vi "select io channels.vi"(8 "error in":errorcluster, 9 "API Loaded":string, 10 "not supported channels":refnum<class "TBM channel.lvclass">[](array[class]), 11 "io channels":refnum<class "TBM channel.lvclass">[](array[class])) -> (0 "error out":errorcluster, 3 "selected channels":refnum<class "TBM channel.lvclass">[](array[class]))   [LabVIEW 2015, in "io editor node.lvclass"]
uses:
  io editor node.lvclass
  <vilib>/NI/Tag Bus Module Framework/channel/TBM channel.lvclass
  table line.ctl
  table reference.ctl
panel:
  in  "Tab Control":enum32{"Static Configuration"}(tab)
  in  "cancel":bool
  in  "select channels":bool
  in  "channel":i32[](listbox)
  out "API Loaded":string
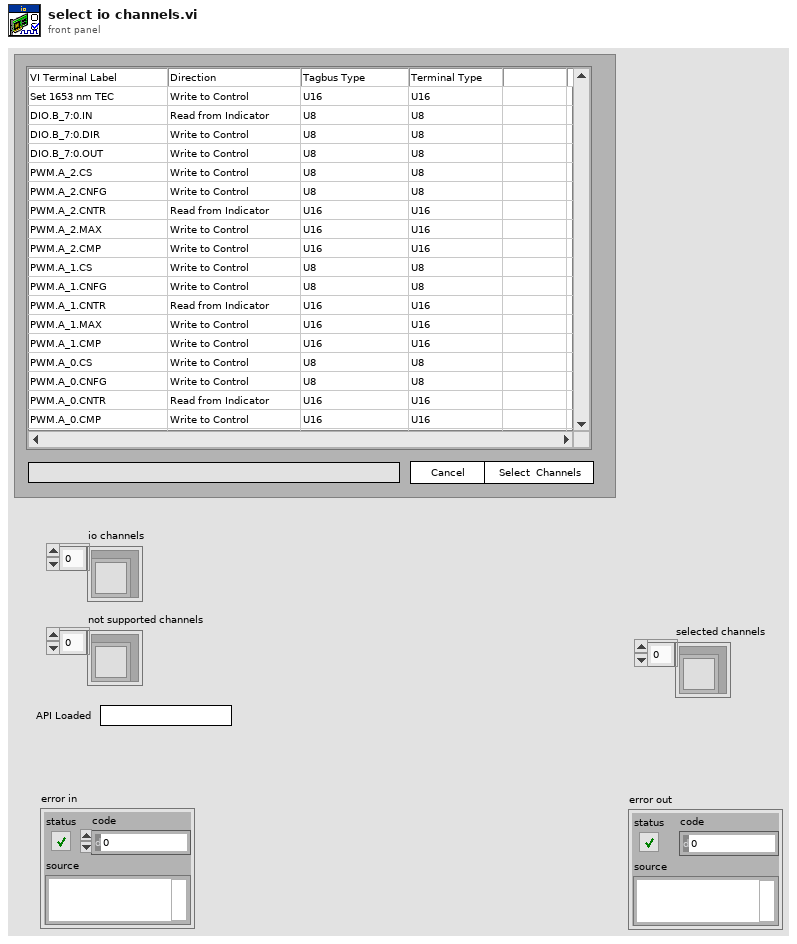
[diagram p1: front panel]
types:
  T1 = typedef "io editor node.lvclass/table line.ctl" = cluster{"channel":refnum<class "TBM channel.lvclass">, "tag name":string}
  T2 = typedef "io editor node.lvclass/table reference.ctl" = refnum<vi>
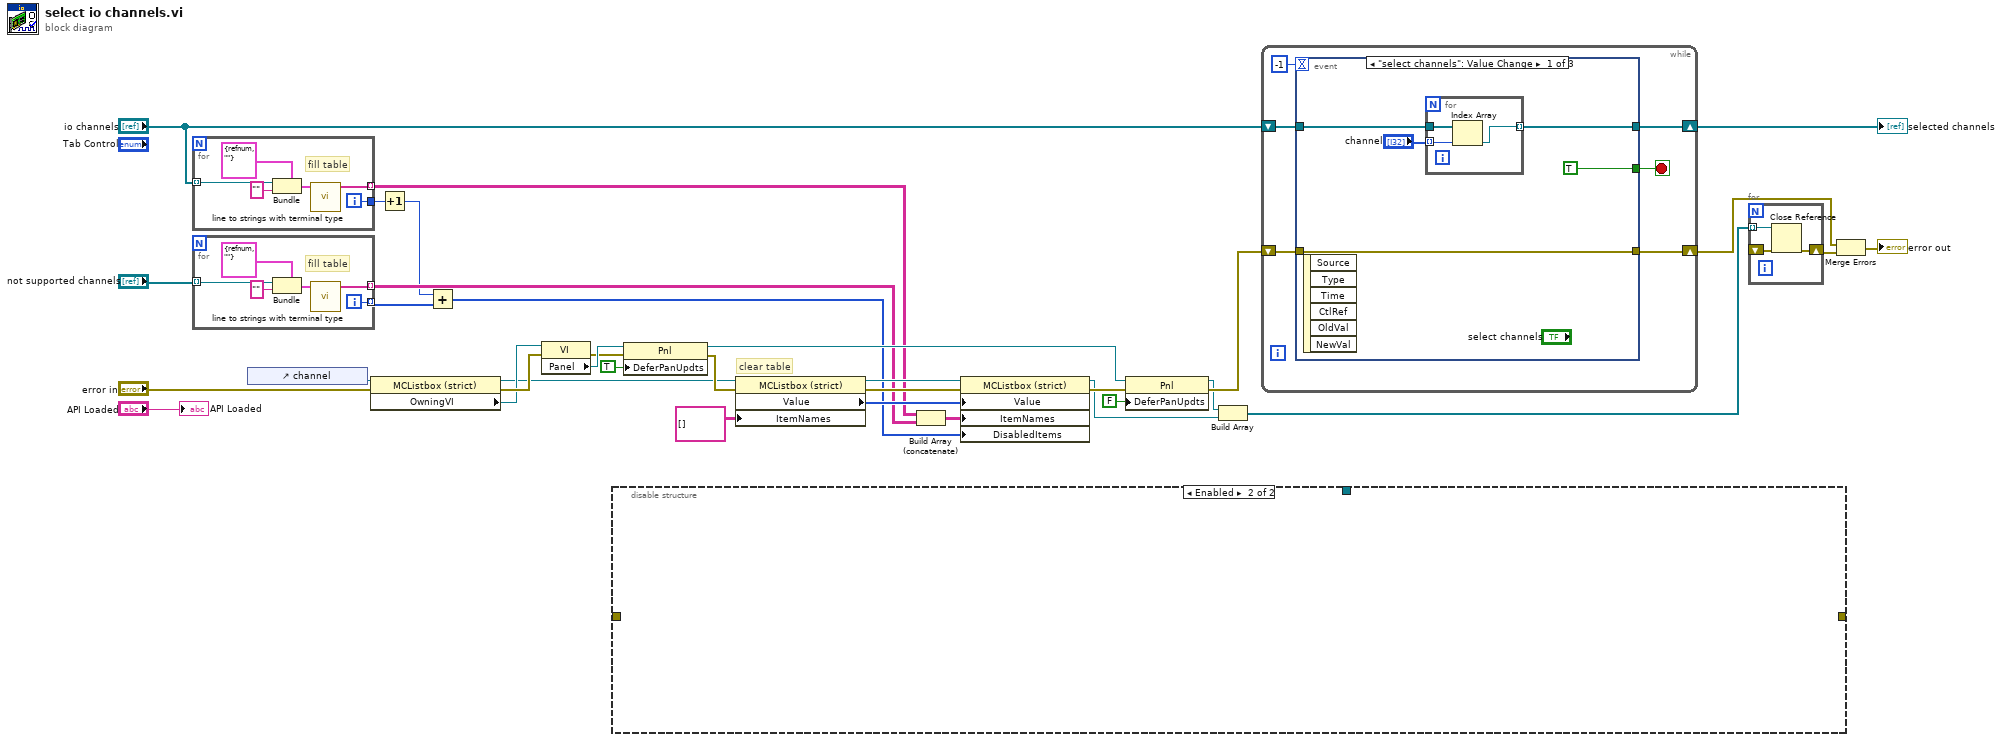
[diagram p0: block diagram]
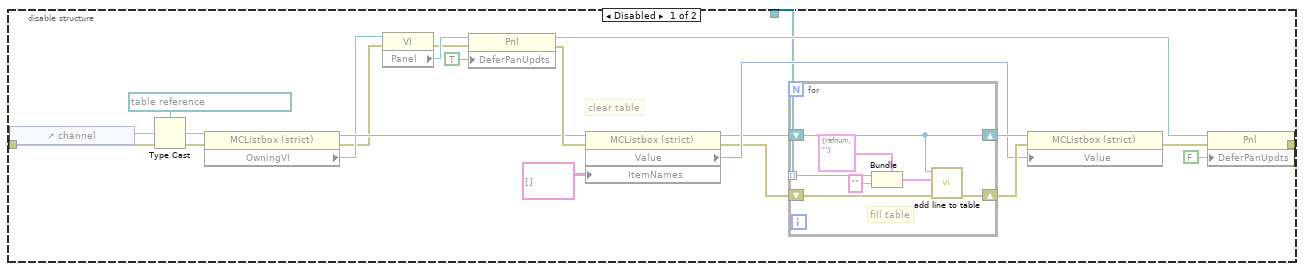
[diagram p2: hidden frame]
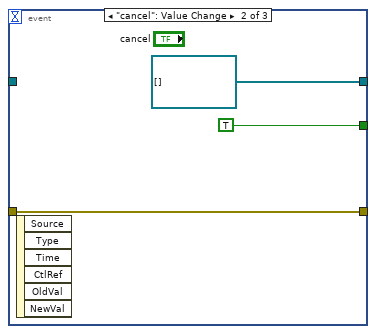
[diagram p3: hidden frame]
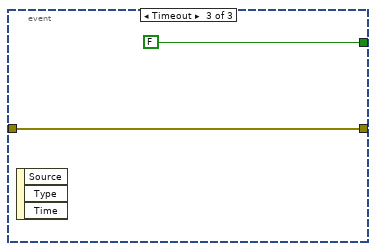
[diagram p4: hidden frame]
diagram:
  # "clear table"
  n1 = for {
    tunnel: "io channels" -> [w39] mode=indexing
    tunnel: [w36] -> w8 mode=indexing
    tunnel: [w35] -> w4
    i -> [w35]
    # "fill table"
    n2 = Bundle(cluster=T1 {"channel"=refnum, "tag name"=""} ("line"), "channel"=w39, "tag name"="") -> (w37:T1)
    n3 = call "line to strings with terminal type.vi"("line"=w37) -> ("strings"=w36:string[])  [unwired: 10 in]
  }
  n4 = for {
    tunnel: "not supported channels" -> [w45] mode=indexing
    tunnel: [w42] -> w6 mode=indexing
    tunnel: [w41] -> w5 mode=indexing
    i -> [w41]
    # "fill table"
    n5 = Bundle(cluster=T1 {"channel"=refnum, "tag name"=""} ("line"), "channel"=w45, "tag name"="") -> (w43:T1)
    n6 = call "line to strings with terminal type.vi"("line"=w43) -> ("strings"=w42:string[])  [unwired: 10 in]
  }
  n7 = control-ref of="channel"() -> (w19:refnum<vi>)
  n8 = property class="MCListbox (strict)"(reference=w19, error in="error in") -> (reference out=w10:refnum<vi>, error out=w20:errorcluster, "OwningVI"=w11:refnum<vi>)
  n9 = Increment(x=w4) -> (x+1=w2:i32)
  n10 = Add(x=w2, y=w5) -> (x+y=w3:i32[])
  n11 = property class="VI"(reference=w11, error in=w20) -> (error out=w24:errorcluster, "Panel"=w25:refnum<vi>)  [unwired: 1 out]
  n12 = disable-structure shown="Enabled" {
    disable-tunnel: _ -> [w49 _]
    disable-tunnel: [w48 _] -> _
    disable-tunnel: _ -> [w47 _]
    frame Disabled {
      # "clear table"
      n13 = control-ref of="channel"() -> (w52:refnum<vi>)
      n14 = Type Cast(type=T2 refnum ("table"), x=w52) -> (*(type *) &x=w51:T2)
      n15 = property class="MCListbox (strict)"(reference=w51, error in=w49) -> (reference out=w57:T2, error out=w55:errorcluster, "OwningVI"=w56:refnum<vi>)
      n16 = property class="VI"(reference=w56, error in=w55) -> (error out=w62:errorcluster, "Panel"=w63:refnum<vi>)  [unwired: 1 out]
      n17 = property class="Pnl"(reference=w63, error in=w62, "DeferPanUpdts"=TRUE ("Defer Panel Updates")) -> (reference out=w59:refnum<vi>, error out=w61:errorcluster)
      n18 = property class="MCListbox (strict)"(reference=w57, error in=w61, "ItemNames"=string[][] [] ("Item Names")) -> (reference out=w53:T2, error out=w54:errorcluster, "Value"=w65:i32)
      n19 = for {
        shift-right: [w75] -> w66
        shift-left: w54 -> [w72]
        shift-right: [w70] -> w67
        shift-left: w53 -> [w70]
        tunnel: w47 -> [w71] mode=indexing
        # "fill table"
        n20 = Bundle(cluster=T1 {"channel"=refnum, "tag name"=""} ("line"), "channel"=w71, "tag name"="") -> (w73:T1)
        n21 = call "add line to table.vi"("error in"=w72, "line"=w73, "operations table"=w70) -> ("error out"=w75:errorcluster)  [unwired: 8 in]
      }
      n22 = property class="MCListbox (strict)"(reference=w67, error in=w66, "Value"=w65) -> (error out=w58:errorcluster)  [unwired: 1 out]
      n23 = property class="Pnl"(reference=w59, error in=w58, "DeferPanUpdts"=FALSE ("Defer Panel Updates")) -> (error out=w48:errorcluster)  [unwired: 1 out]
    }
    frame Enabled {
    }
  }
  n24 = property class="Pnl"(reference=w25, error in=w24, "DeferPanUpdts"=TRUE ("Defer Panel Updates")) -> (reference out=w21:refnum<vi>, error out=w23:errorcluster)
  n25 = property class="MCListbox (strict)"(reference=w10, error in=w23, "ItemNames"=string[][] [] ("Item Names")) -> (reference out=w18:refnum<vi>, error out=w17:errorcluster, "Value"=w27:i32[])
  n26 = Build Array (concatenate)(w8, w6) -> (w7:string[][])
  n27 = property class="MCListbox (strict)"(reference=w18, error in=w17, "Value"=w27, "ItemNames"=w7, "DisabledItems"=w3) -> (reference out=w14:refnum<vi>, error out=w16:errorcluster)
  n28 = property class="Pnl"(reference=w21, error in=w16, "DeferPanUpdts"=FALSE ("Defer Panel Updates")) -> (reference out=w15:refnum<vi>, error out=w34:errorcluster)
  n29 = Build Array(w15, w14) -> (w32:refnum<vi>[])
  n30 = while {
    shift-right: [w77] -> w30
    shift-left: w34 -> [w78]
    shift-right: [w80] -> w1
    shift-left: "io channels" -> [w81]
    stop <- w79 stop-if-true
    n31 = event shown="[0] \"select channels\": Value Change" {
      selector: _ -> [_ _ _]
      dyn-events: _ -> [_ _ _]
      timeout: -1 -> [_ _ _]
      tunnel: w81 -> [w84 _ _]
      tunnel: [w83 refnum<class "TBM channel.lvclass">[] [] ("selected channels") _] -> w80
      tunnel: [TRUE TRUE FALSE] -> w79
      tunnel: w78 -> [w86 w90 w94]
      tunnel: [w86 w90 w94] -> w77
      event "select channels": Value Change {
        n32 = event-data() -> ()  [unwired: 1 in, 6 out]
        n33 = for {
          tunnel: "channel" -> [w89] mode=indexing
          tunnel: w84 -> [w88]
          tunnel: [w87] -> w83 mode=indexing
          n34 = Index Array(array=w88, index=w89) -> (element=w87:refnum<class "TBM channel.lvclass">)
        }
      }
      event "cancel": Value Change {
        n35 = event-data() -> ()  [unwired: 1 in, 6 out]
      }
      event Timeout {
        n36 = event-data() -> ()  [unwired: 1 in, 3 out]
      }
    }
  }
  "selected channels" <- w1
  n37 = for {
    shift-right: [w96] -> w31
    shift-left: _ -> [w97]
    tunnel: w32 -> [w95] mode=indexing
    n38 = Close Reference(reference=w95, error in (no error)=w97) -> (error out=w96:errorcluster)
  }
  n39 = Merge Errors(w30, w31) -> (→"error out":errorcluster)
  "API Loaded" <- "API Loaded"
